vi "Get Event Timing Captures.vi"(0 "Item Ref in":T2 format="%.0x", 1 "Window":string, 5 "Timing measurement":string, 7 "return all captures (T)":bool=TRUE, 11 "error in (no error)":errorcluster) -> (2 "window":T1, 3 "not present indexes":i32[](array[numeric]), 4 "Item Ref out":T2 format="%.0x", 6 "captures":T3[](array[typedef]), 8 "window found":bool, 10 "Window reference angle":dbl, 12 "Capture item refs":T2[](array[typedef]) format="%.0x", 14 "degrees of one u16":dbl, 15 "error out":errorcluster)   [LabVIEW 2015, in "Engine Simulation Toolkit System Explorer.lvlib"]
uses:
  Engine Simulation Toolkit System Explorer.lvlib
  Event Timing Capture.ctl
  Event Reference Angle Selection.ctl
  <vilib>/NI Veristand/Custom Device API/Custom Device Item Ref.ctl
  Event Timing Window.ctl
  Shared/Properties.vi
  Shared/Constants and GUIDs.vi
  <vilib>/NI Veristand/Custom Device Tools/Custom Device Utility Library/NI VeriStand - Search for All Items by GUID.vi
  <vilib>/NI Veristand/Custom Device API/Get Item Property (String).vi
  <vilib>/NI Veristand/Custom Device API/Get Item Property (Double).vi
  <vilib>/NI Veristand/Custom Device API/Get Item Property (U16).vi
  Shared/Engine Simulation Toolkit Shared.lvlib
  <vilib>/NI Veristand/Custom Device API/Custom Device API.lvlib
  <vilib>/NI Veristand/Custom Device Tools/Custom Device Utility Library/Custom Device Utility Library.lvlib
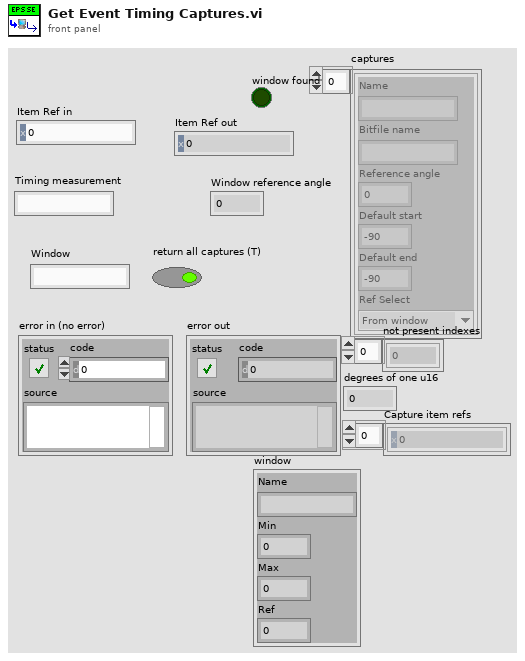
[diagram p1: front panel]
types:
  T1 = typedef "Engine Simulation Toolkit System Explorer.lvlib/Event Timing Window.ctl" = cluster{"Name":string, "Min":dbl, "Max":dbl, "Ref":dbl}
  T2 = typedef "Custom Device API.lvlib/Custom Device Item Ref.ctl" = u64
  T3 = typedef "Engine Simulation Toolkit System Explorer.lvlib/Event Timing Capture.ctl" = cluster{"Name":string, "Bitfile name":string, "Reference angle":dbl, "Default start":dbl, "Default end":dbl, "Ref Select":T4}
  T4 = typedef "Engine Simulation Toolkit System Explorer.lvlib/Event Reference Angle Selection.ctl" = enum16{"From window", "Custom"}
  T5 = typedef "Custom Device API.lvlib/Custom Device Item Info.ctl" = cluster{"Name":string, "Is Channel":bool, "GUID":string, "Is Waveform":bool}
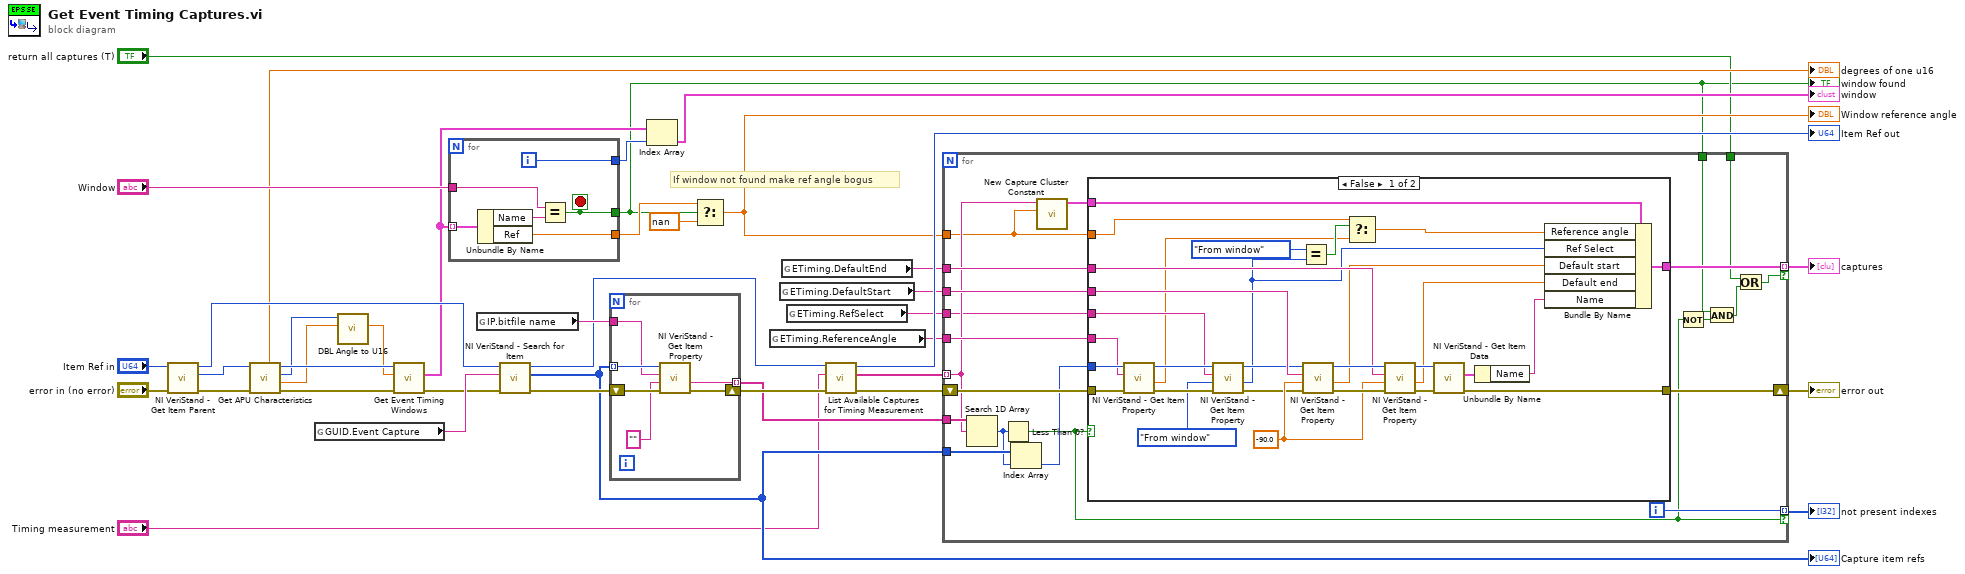
[diagram p0: block diagram]
diagram:
  # "If window not found make ref angle bogus"
  n1 = call <vilib>:"NI VeriStand - Get Item Parent.vi"("error in (no error)"="error in (no error)", "Item Ref in"="Item Ref in") -> ("error out"=w15:errorcluster, "Parent Ref"=w14:T2, "Item Ref out"=w11:T2)  [unwired: 6 in, 1 out]
  n2 = call "Get APU Characteristics.vi"("error in (no error)"=w15, "Item Ref in"=w14) -> ("error out"=w20:errorcluster, "angle to u16 scale factor"=w16:dbl, "total angle span (degrees)"=w17:u16, "Item Ref out"=w19:T2, "degrees of one u16"=→"degrees of one u16":dbl)  [unwired: 3 in, 2 out]
  n3 = global read "Constants and GUIDs.vi" "GUID.Event Capture"() -> (w22:string)
  n4 = call "DBL Angle to U16.vi"("angle to u16 scale factor"=w16, "Desired angle (degrees)"=w17) -> ("Actual angle (degrees)"=w18:dbl)  [unwired: 8 in, 1 out]
  n5 = call "Get Event Timing Windows.vi"("error in (no error)"=w20, "Max engine angle"=w18, "Item Ref in"=w19) -> ("error out"=w13:errorcluster, "Windows"=w5:T1[])  [unwired: 6 in, 1 out]
  n6 = for {
    tunnel: w5 -> [w45] mode=indexing
    tunnel: "Window" -> [w43]
    tunnel: [w42] -> w9
    tunnel: [w41] -> w1
    tunnel: [w40] -> w4
    i -> [w40]
    stop <- w41 stop-if-true
    n7 = Unbundle By Name(w45) -> ("Name"=w44:string, "Ref"=w42:dbl)
    n8 = Equal?(x=w43, y=w44) -> (x = y?=w41:bool)
  }
  "window found" <- w1
  n9 = global read "Properties.vi" "IP.bitfile name"() -> (w29:string)
  n10 = call-poly <vilib>:"NI VeriStand - Search for Item.vi"("error in"=w13, "Item GUID"=w22, "Section Ref in"=w11) -> ("error out"=w30:errorcluster, "Item Refs"=w25:T2[], "Section Ref out"=w28:T2)  [unwired: 5 in, 1 out]
  "Capture item refs" <- w25
  n11 = for {
    shift-right: [w48] -> w27
    shift-left: w30 -> [w51]
    tunnel: w25 -> [w50] mode=indexing
    tunnel: w29 -> [w49]
    tunnel: [w46] -> w26 mode=indexing
    n12 = call-poly <vilib>:"NI VeriStand - Get Item Property.vi"("error in (no error)"=w51, "Default Value"="", "Property Name"=w49, "Item Ref in"=w50) -> ("error out"=w48:errorcluster, "Value"=w46:string)  [unwired: 4 in, 2 out]
  }
  n13 = Index Array(array=w5, index=w4) -> (element=→"window":T1)
  n14 = Select(t=w9, s=w1, f=nan) -> (s? t:f=w7:dbl)
  "Window reference angle" <- w7
  n15 = global read "Properties.vi" "ETiming.ReferenceAngle"() -> (w33:string)
  n16 = global read "Properties.vi" "ETiming.DefaultStart"() -> (w32:string)
  n17 = global read "Properties.vi" "ETiming.DefaultEnd"() -> (w24:string)
  n18 = global read "Properties.vi" "ETiming.RefSelect"() -> (w10:string)
  n19 = call "List Available Captures for Timing Measurement.vi"("error in (no error)"=w27, "Timing measurement"="Timing measurement", "Item Ref in"=w28) -> ("error out"=w37:errorcluster, "captures available"=w36:string[], "Item Ref out"=→"Item Ref out":T2)  [unwired: 6 in]
  n20 = for {
    tunnel: [w60] -> w39 mode=indexing if=w57
    shift-right: [w70] -> w34
    shift-left: w37 -> [w68]
    tunnel: w36 -> [w61] mode=indexing
    tunnel: w33 -> [w72]
    tunnel: w32 -> [w71]
    tunnel: [w69] -> w31 mode=indexing if=w54
    tunnel: w26 -> [w67]
    tunnel: w25 -> [w66]
    tunnel: w24 -> [w63]
    tunnel: w10 -> [w59]
    tunnel: w7 -> [w58]
    tunnel: "return all captures (T)" -> [w56]
    tunnel: w1 -> [w52]
    i -> [w69]
    n21 = Search 1D Array(1D array=w67, element=w61) -> (index of element=w65:i32)  [unwired: 1 in]
    n22 = Less Than 0?(x=w65) -> (x < 0?=w54:bool)
    n23 = Index Array(array=w66, index=w65) -> (element=w64:T2)
    n24 = call "New Capture Cluster Constant.vi"("Window ref angle"=w58, "Bitfile name"=w61) -> ("Capture"=w62:T3)  [unwired: 9 in]
    n25 = case shown="False" w54 {
      tunnel: w68 -> [w101 w103]
      tunnel: w64 -> [w100 _]
      tunnel: w72 -> [w99 _]
      tunnel: w71 -> [w97 _]
      tunnel: [w95 w103] -> w70
      tunnel: w63 -> [w90 _]
      tunnel: w62 -> [w89 w102]
      tunnel: [w85 w102] -> w60
      tunnel: w59 -> [w80 _]
      tunnel: w58 -> [w75 _]
      frame False {
        w84 = -90.0
        n26 = call-poly <vilib>:"NI VeriStand - Get Item Property.vi"("error in (no error)"=w101, "Property Name"=w99, "Item Ref in"=w100) -> ("error out"=w98:errorcluster, "Value"=w76:dbl, "Item Ref out"=w82:T2)  [unwired: 5 in, 1 out]
        n27 = call-poly <vilib>:"NI VeriStand - Get Item Property.vi"("error in (no error)"=w98, "Default Value"=Event_Reference_Angle_Selection."From window" ("Reference angle"), "Property Name"=w80, "Item Ref in"=w82) -> ("error out"=w83:errorcluster, "Value"=w73:u16, "Item Ref out"=w81:T2)  [unwired: 4 in, 1 out]
        n28 = Equal?(x=Event_Reference_Angle_Selection."From window" ("Reference angle"), y=w73) -> (x = y?=w77:bool)
        n29 = call-poly <vilib>:"NI VeriStand - Get Item Property.vi"("error in (no error)"=w83, "Default Value"=w84, "Property Name"=w97, "Item Ref in"=w81) -> ("error out"=w96:errorcluster, "Value"=w88:dbl, "Item Ref out"=w92:T2)  [unwired: 4 in, 1 out]
        n30 = Select(t=w75, s=w77, f=w76) -> (s? t:f=w74:dbl)
        n31 = call-poly <vilib>:"NI VeriStand - Get Item Property.vi"("error in (no error)"=w96, "Default Value"=w84, "Property Name"=w90, "Item Ref in"=w92) -> ("error out"=w93:errorcluster, "Value"=w87:dbl, "Item Ref out"=w91:T2)  [unwired: 4 in, 1 out]
        n32 = call <vilib>:"NI VeriStand - Get Item Data.vi"("error in (no error)"=w93, "Item Ref in"=w91) -> ("error out"=w95:errorcluster, "Item Info"=w94:T5)  [unwired: 6 in, 2 out]
        n33 = Unbundle By Name(w94) -> ("Name"=w86:string)
        n34 = Bundle By Name(cluster=w89, "Reference angle"=w74, "Ref Select"=w73, "Default start"=w88, "Default end"=w87, "Name"=w86) -> (w85:T3)
      }
      frame True {
      }
    }
    n35 = Not(x=w54) -> (.not. x?=w55:bool)
    n36 = And(x=w52, y=w55) -> (x .and. y?=w53:bool)
    n37 = Or(x=w56, y=w53) -> (x .or. y?=w57:bool)
  }
  "error out" <- w34
  "captures" <- w39
  "not present indexes" <- w31
